vi "JJMCclase4.vi"() -> ()   [LabVIEW 2011]
panel:
  out "Alarma":bool
  out "Thermometer":dbl(slide) scale=0.0..100.0
  out "Cambio":string
  out "Cuarta":bool
  out "Tercera":bool
  out "Segunda":bool
  out "Primera":bool
  out "Velocidad":i32(knob) scale=0.0..180.0
  # "elaborar un programa donde se genere la velocidad entre 1-180, luego de acuerdo a la velocidad que se alcance \nencender que cambio se encuentra y escribir en el string el cambio\n1-40 primera\n41-60 segunda\n61-80 tercera\n81-180 cuarta\nSi la temp es mayor a 75 y  la velocidad mayor a 120 encender alarma"
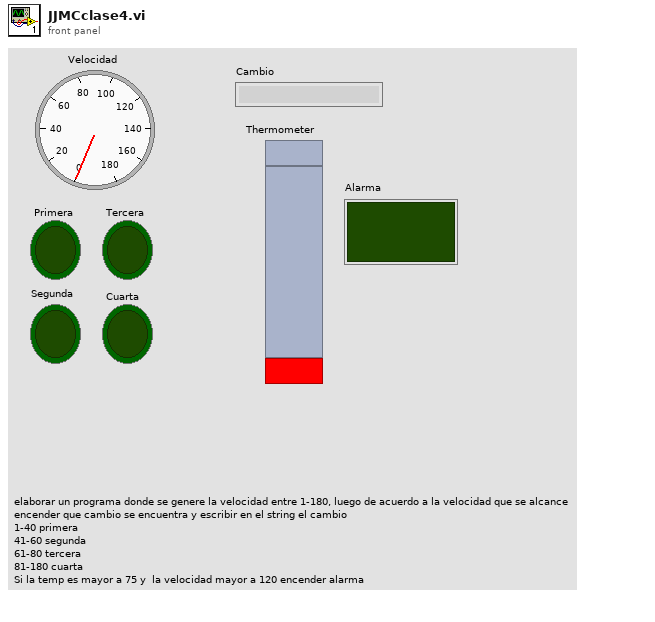
[diagram p1: front panel]
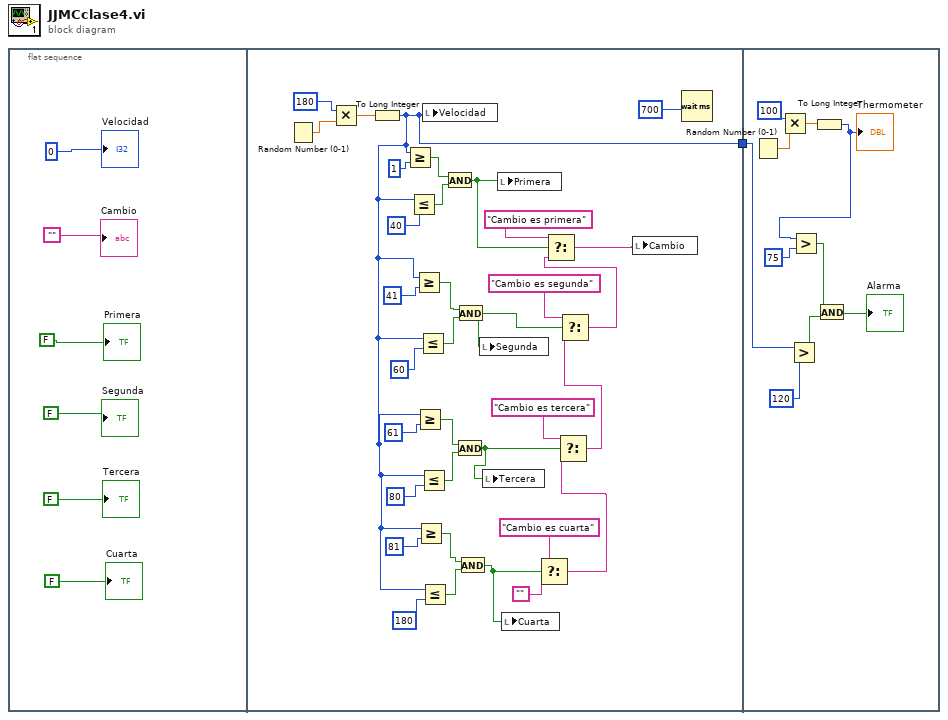
[diagram p0: block diagram]
diagram:
  n1 = flat-sequence {
    tunnel: [w8] -> w1
    tunnel: w1 -> [w42]
    frame #0 {
      "Velocidad" <- 0
      "Primera" <- FALSE
      "Segunda" <- FALSE
      "Tercera" <- FALSE
      "Cuarta" <- FALSE
      "Cambio" <- ""
    }
    frame #1 {
      n2 = Random Number (0-1)() -> (number: 0 to 1=w39:dbl)
      n3 = Multiply(x=180, y=w39) -> (x*y=w41:dbl)
      n4 = To Long Integer(number=w41) -> (32bit integer=w8:i32)
      n5 = Greater Or Equal?(x=w8, y=1) -> (x >= y?=w36:bool)
      n6 = Less Or Equal?(x=w8, y=40) -> (x <= y?=w35:bool)
      n7 = Greater Or Equal?(x=w8, y=41) -> (x >= y?=w28:bool)
      n8 = Greater Or Equal?(x=w8, y=61) -> (x >= y?=w21:bool)
      n9 = Greater Or Equal?(x=w8, y=81) -> (x >= y?=w19:bool)
      n10 = Less Or Equal?(x=w8, y=60) -> (x <= y?=w29:bool)
      n11 = Less Or Equal?(x=w8, y=80) -> (x <= y?=w22:bool)
      n12 = Less Or Equal?(x=w8, y=180) -> (x <= y?=w20:bool)
      n13 = local write "Velocidad"(w8) -> ()
      n14 = And(x=w36, y=w35) -> (x .and. y?=w30:bool)
      n15 = And(x=w21, y=w22) -> (x .and. y?=w12:bool)
      n16 = And(x=w28, y=w29) -> (x .and. y?=w13:bool)
      n17 = And(x=w19, y=w20) -> (x .and. y?=w10:bool)
      n18 = local write "Segunda"(w13) -> ()
      n19 = local write "Tercera"(w12) -> ()
      n20 = local write "Primera"(w30) -> ()
      n21 = local write "Cuarta"(w10) -> ()
      n22 = Select(t="Cambio es cuarta", s=w10, f="") -> (s? t:f=w11:string)
      n23 = Select(t="Cambio es tercera", s=w12, f=w11) -> (s? t:f=w14:string)
      n24 = Select(t="Cambio es segunda", s=w13, f=w14) -> (s? t:f=w18:string)
      n25 = Select(t="Cambio es primera", s=w30, f=w18) -> (s? t:f=w31:string)
      n26 = local write "Cambio"(w31) -> ()
      n27 = Wait (ms)(milliseconds to wait=700) -> ()  [unwired: 1 out]
    }
    frame #2 {
      n28 = Random Number (0-1)() -> (number: 0 to 1=w47:dbl)
      n29 = Multiply(x=100, y=w47) -> (x*y=w46:dbl)
      n30 = Greater?(x=w42, y=120) -> (0:w49:bool)
      n31 = To Long Integer(number=w46) -> (32bit integer=w44:i32)
      "Thermometer" <- w44
      n32 = Greater?(x=w44, y=75) -> (0:w50:bool)
      "Alarma" <- w50
      n33 = And(x=w50, y=w49) -> ()  [unwired: 1 out]
    }
  }
